vi "subCalculate_DisableScaleBar.vi"(8 "Total y width in (μm)":refnum<vi>, 9 "Total x width in (μm)":refnum<vi>, 10 "Distance per pixel (nm)":refnum<vi>, 11 "measuring scale (μm)":refnum<vi>) -> ()   [LabVIEW 2015]
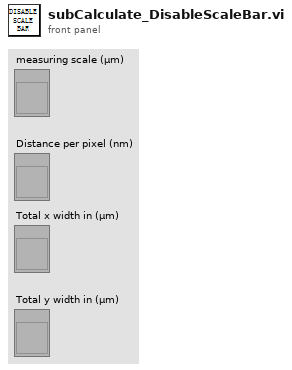
[diagram p1: front panel]
types:
  T1 = enum8{"Enabled", "Disabled", "Disabled and Grayed Out"}
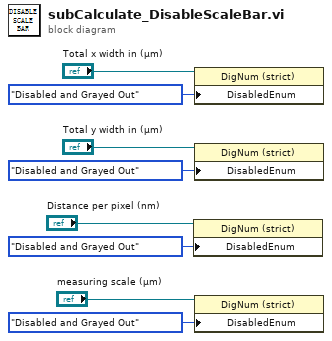
[diagram p0: block diagram]
diagram:
  n1 = property class="DigNum (strict)"(reference="Distance per pixel (nm)", "DisabledEnum"=T1."Disabled and Grayed Out" ("Disabled")) -> ()  [unwired: 1 in, 2 out]
  n2 = property class="DigNum (strict)"(reference="Total x width in (μm)", "DisabledEnum"=T1."Disabled and Grayed Out" ("Disabled")) -> ()  [unwired: 1 in, 2 out]
  n3 = property class="DigNum (strict)"(reference="Total y width in (μm)", "DisabledEnum"=T1."Disabled and Grayed Out" ("Disabled")) -> ()  [unwired: 1 in, 2 out]
  n4 = property class="DigNum (strict)"(reference="measuring scale (μm)", "DisabledEnum"=T1."Disabled and Grayed Out" ("Disabled")) -> ()  [unwired: 1 in, 2 out]
